vi "delta.vi"(1 "c":dbl=2.0, 2 "b":dbl=3.0, 3 "a":dbl=1.0) -> (0 "delta":dbl=1.0)   [LabVIEW 2021]
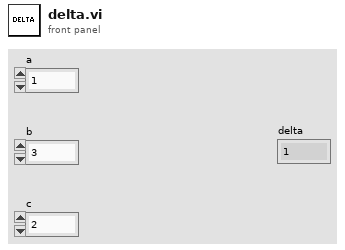
[diagram p1: front panel]
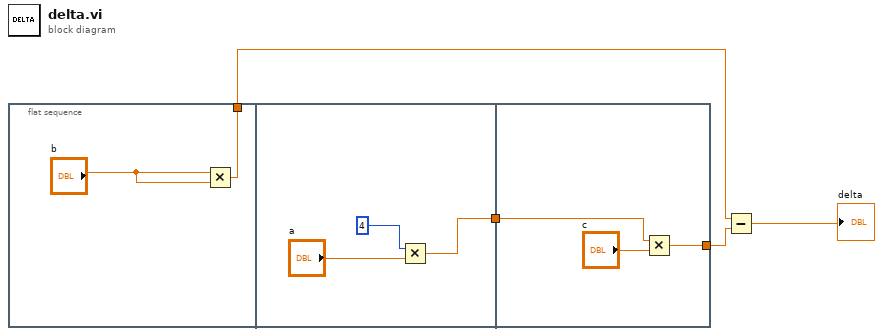
[diagram p0: block diagram]
diagram:
  n1 = flat-sequence {
    tunnel: [w5] -> w3
    tunnel: [w7] -> w2
    tunnel: w2 -> [w11]
    tunnel: [w10] -> w1
    frame #0 {
      n2 = Multiply(x="b", y="b") -> (x*y=w5:dbl)
    }
    frame #1 {
      n3 = Multiply(x=4, y="a") -> (x*y=w7:dbl)
    }
    frame #2 {
      n4 = Multiply(x=w11, y="c") -> (x*y=w10:dbl)
    }
  }
  n5 = Subtract(x=w3, y=w1) -> (x-y=→"delta":dbl)
